vi "Acquire.vi"(8 "error in (no error)":errorcluster, 11 "ATS9462 Class in":refnum<class "ATS9462 Class.lvclass">) -> (0 "error out":errorcluster, 3 "ATS9462 Class out":refnum<class "ATS9462 Class.lvclass">)   [LabVIEW 2014, in "ATS9462 Class.lvclass"]
uses:
  ATS9462 Class.lvclass
  ATS-VI/ATS_ctl/ATS_Async_Ctrl.ctl
  DAQ Control Functional Global States.ctl
  DAQ Status States.ctl
  DAQ Class.lvclass
panel:
  out "Reset DAQ":bool
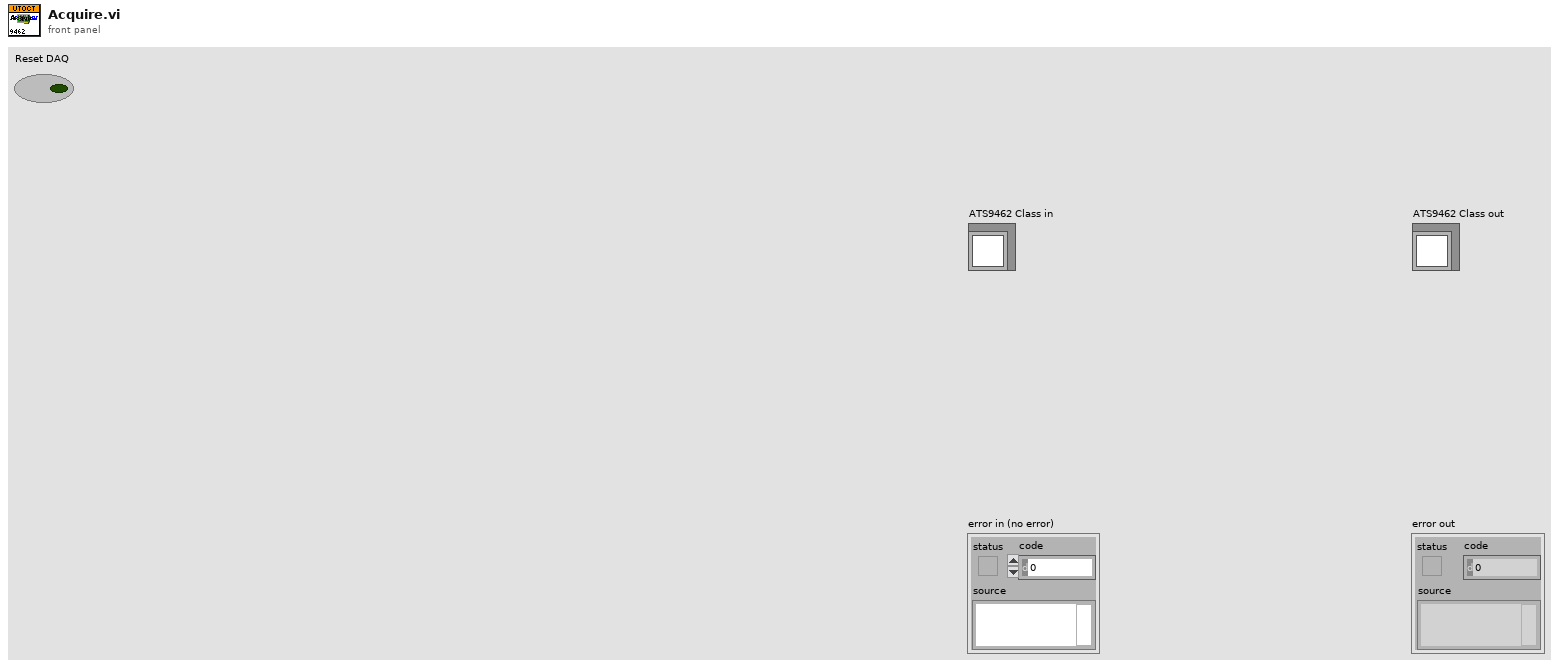
[diagram p1: front panel]
types:
  T1 = typedef "DAQ Control Functional Global States.ctl" = enum16{"Status", "Set Processing Finished", "Reset", "Clear", "Set DAQ Finished"}
  T2 = typedef "ATS_Async_Ctrl.ctl" = enum16{"SetupDMA", "StartCapture", "Get", "Get_Stream", "Abort", "Stop"}
  T3 = typedef "DAQ Status States.ctl" = enum16{"Get", "Show"}
  T4 = typedef "ATS_Async_Status.ctl" = cluster{"Start DMA":bool, "StartCapture":bool, "Valid":bool, "Completed":bool, "InProgress":bool, "Timeout":bool, "Overflow":bool, "Error":bool}
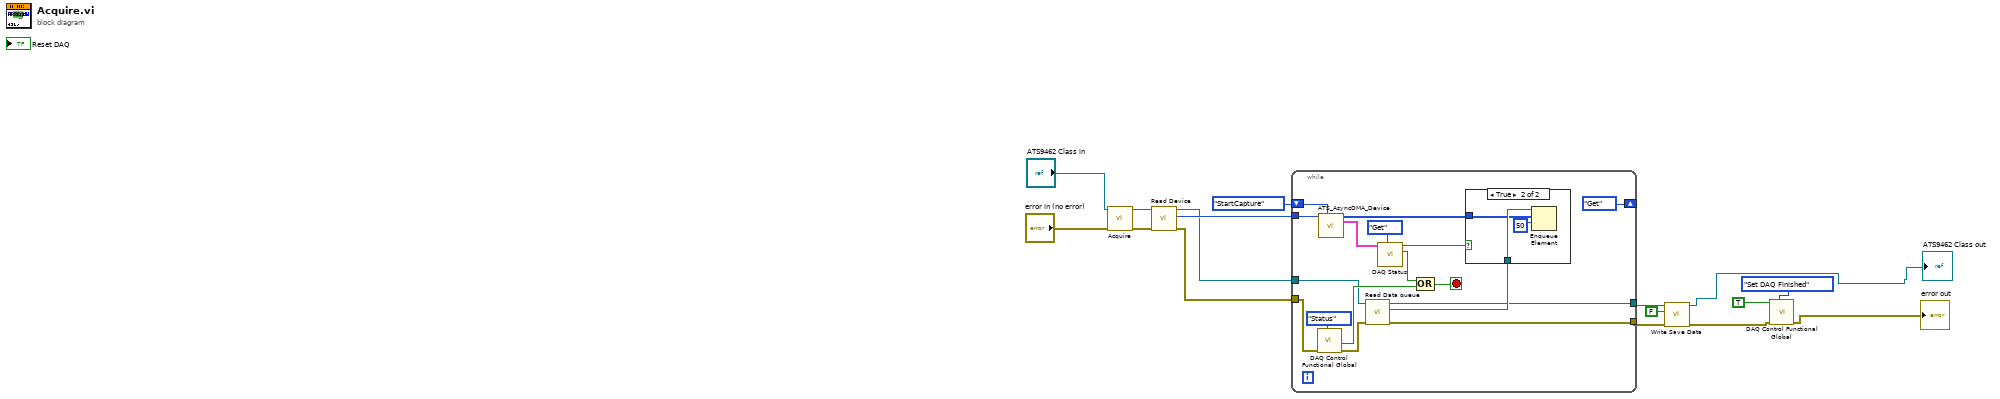
[diagram p0: block diagram]
diagram:
  n1 = call-parent "Acquire.vi"("error in (no error)"="error in (no error)", "DAQ Class in"="ATS9462 Class in") -> ("error out"=w14:errorcluster, "DAQ Class out"=w13:refnum<class "ATS9462 Class.lvclass">)  [unwired: 8 in]
  n2 = call-dynamic "Read Device.vi"("error in (no error)"=w14, "ATS9462 Class in"=w13) -> ("error out"=w7:errorcluster, "Device"=w12:i32, "ATS9462 Class out"=w8:refnum<class "ATS9462 Class.lvclass">)  [unwired: 7 in]
  n3 = while {
    tunnel: w12 -> [w33]
    shift-right: [ATS_Async_Ctrl."Get" ("ATS_Async_Ctrl")] -> _
    shift-left: ATS_Async_Ctrl."StartCapture" ("ATS_Async_Ctrl") -> [w32]
    tunnel: w8 -> [w18]
    tunnel: w7 -> [w19]
    tunnel: [w24] -> w5
    tunnel: [w23] -> w4
    stop <- w29 stop-if-true
    n4 = call "DAQ Control Functional Global.vi"("State"=DAQ_Control_Functional_Global_States."Status", "Error In"=w19) -> ("Error Out"=w21:errorcluster, "Reset?"=w20:bool)  [unwired: 6 in, 2 out]
    n5 = call "ATS_AsyncDMA_Device.vi"("DeviceIn"=w33, "ATS_Async_Ctrl"=w32) -> ("Buffer"=w30:u16[], "Async_Status"=w28:T4)  [unwired: 9 in, 3 out]
    n6 = call-dynamic "Read Data queue.vi"("error in (no error)"=w21, "DAQ Class in"=w18) -> ("error out"=w24:errorcluster, "Data queue"=w25:refnum<queue>, "DAQ Class out"=w23:refnum<class "ATS9462 Class.lvclass">)  [unwired: 7 in]
    n7 = call "DAQ Status.vi"("Enum"=DAQ_Status_States."Get", "Async_Status"=w28) -> ("DAQ Error?"=w17:bool, "Valid"=w27:bool)  [unwired: 8 in]
    n8 = Compound Arithmetic op=OR(w17, w20) -> (w29:bool)
    n9 = case shown="True" w27 {
      tunnel: w30 -> [_ w34]
      tunnel: w25 -> [_ w36]
      frame False {
        # "Do nothing"
      }
      frame True {
        n10 = Enqueue Element(queue=w36, element=w34, timeout in ms (-1)=50) -> ()  [unwired: 1 in, 3 out]
      }
    }
  }
  n11 = call-dynamic "Write Save Data.vi"("error in (no error)"=w5, "Save Data"=FALSE, "DAQ Class in"=w4) -> ("error out"=w2:errorcluster, "DAQ Class out"=→"ATS9462 Class out":refnum<class "ATS9462 Class.lvclass">)  [unwired: 7 in]
  n12 = call "DAQ Control Functional Global.vi"("State"=DAQ_Control_Functional_Global_States."Set DAQ Finished", "Error In"=w2, "DAQ Finished In"=TRUE) -> ("Error Out"=→"error out":errorcluster)  [unwired: 5 in, 3 out]
